vi "Incorporate New Data.vi"(8 "error in (no error)":cluster{"状态":bool, "代码":i32, "源":string} caption="错误输入（无错误）", 10 "新图形数据":waveform(dbl)[](array[waveform]), 11 "数据输入":T1={"UI引用"={"退出引用"=refnum, "保存引用"=refnum, "打开引用"=refnum, "导出引用"=refnum, "采集引用"=refnum, "配置引用"=refnum, "图形引用"=refnum, "清空引用"=refnum, "分析引用"=refnum, "状态引用"=refnum, "快照引用"=refnum}, "图形数据"={"数据"=[], "注释列表"=[], "游标列表"=[], "分析数据"=[]}, "用户定义"={"硬件配置"={"硬件引用句柄<替换此项>"="", "信号类型<替换该项>"=enum."Sine Wave"}, "分析配置"={"统计"=TRUE}, "新采集到数据时如何操作"=enum."Replace"}}) -> (0 "error out":cluster{"状态":bool, "代码":i32, "源":string} caption="错误输出", 3 "数据输出":T1={"UI引用"={"退出引用"=refnum, "保存引用"=refnum, "打开引用"=refnum, "导出引用"=refnum, "采集引用"=refnum, "配置引用"=refnum, "图形引用"=refnum, "清空引用"=refnum, "分析引用"=refnum, "状态引用"=refnum, "快照引用"=refnum}, "图形数据"={"数据"=[], "注释列表"=[], "游标列表"=[], "分析数据"=[]}, "用户定义"={"硬件配置"={"硬件引用句柄<替换此项>"="", "信号类型<替换该项>"=enum."Sine Wave"}, "分析配置"={"统计"=TRUE}, "新采集到数据时如何操作"=enum."Replace"}})   [LabVIEW 2022 SP3]
doc: "将新采集到的数据或加载的数据与主状态数据整合。 新数据可以替换、追加，或与原有数据重叠（作为额外的通道）。 如尚无保存好的用户配置，将会弹出对话框询问用户。"
uses:
  controls/Data.ctl
  controls/UI References.ctl
  controls/Graph Data.ctl
  <vilib>/Utility/miscctls.llb/LVAnnotationListTypeDef.ctl
  <vilib>/Utility/miscctls.llb/LVCursorListTypeDef.ctl
  controls/User Specified Data.ctl
  controls/HW Configuration.ctl
  controls/Simulated Signal Type.ctl
  controls/Analysis Configuration.ctl
  controls/New Data Behavior.ctl
panel:
  # "（向上滚动可查看大型状态数据输入/输出簇）"
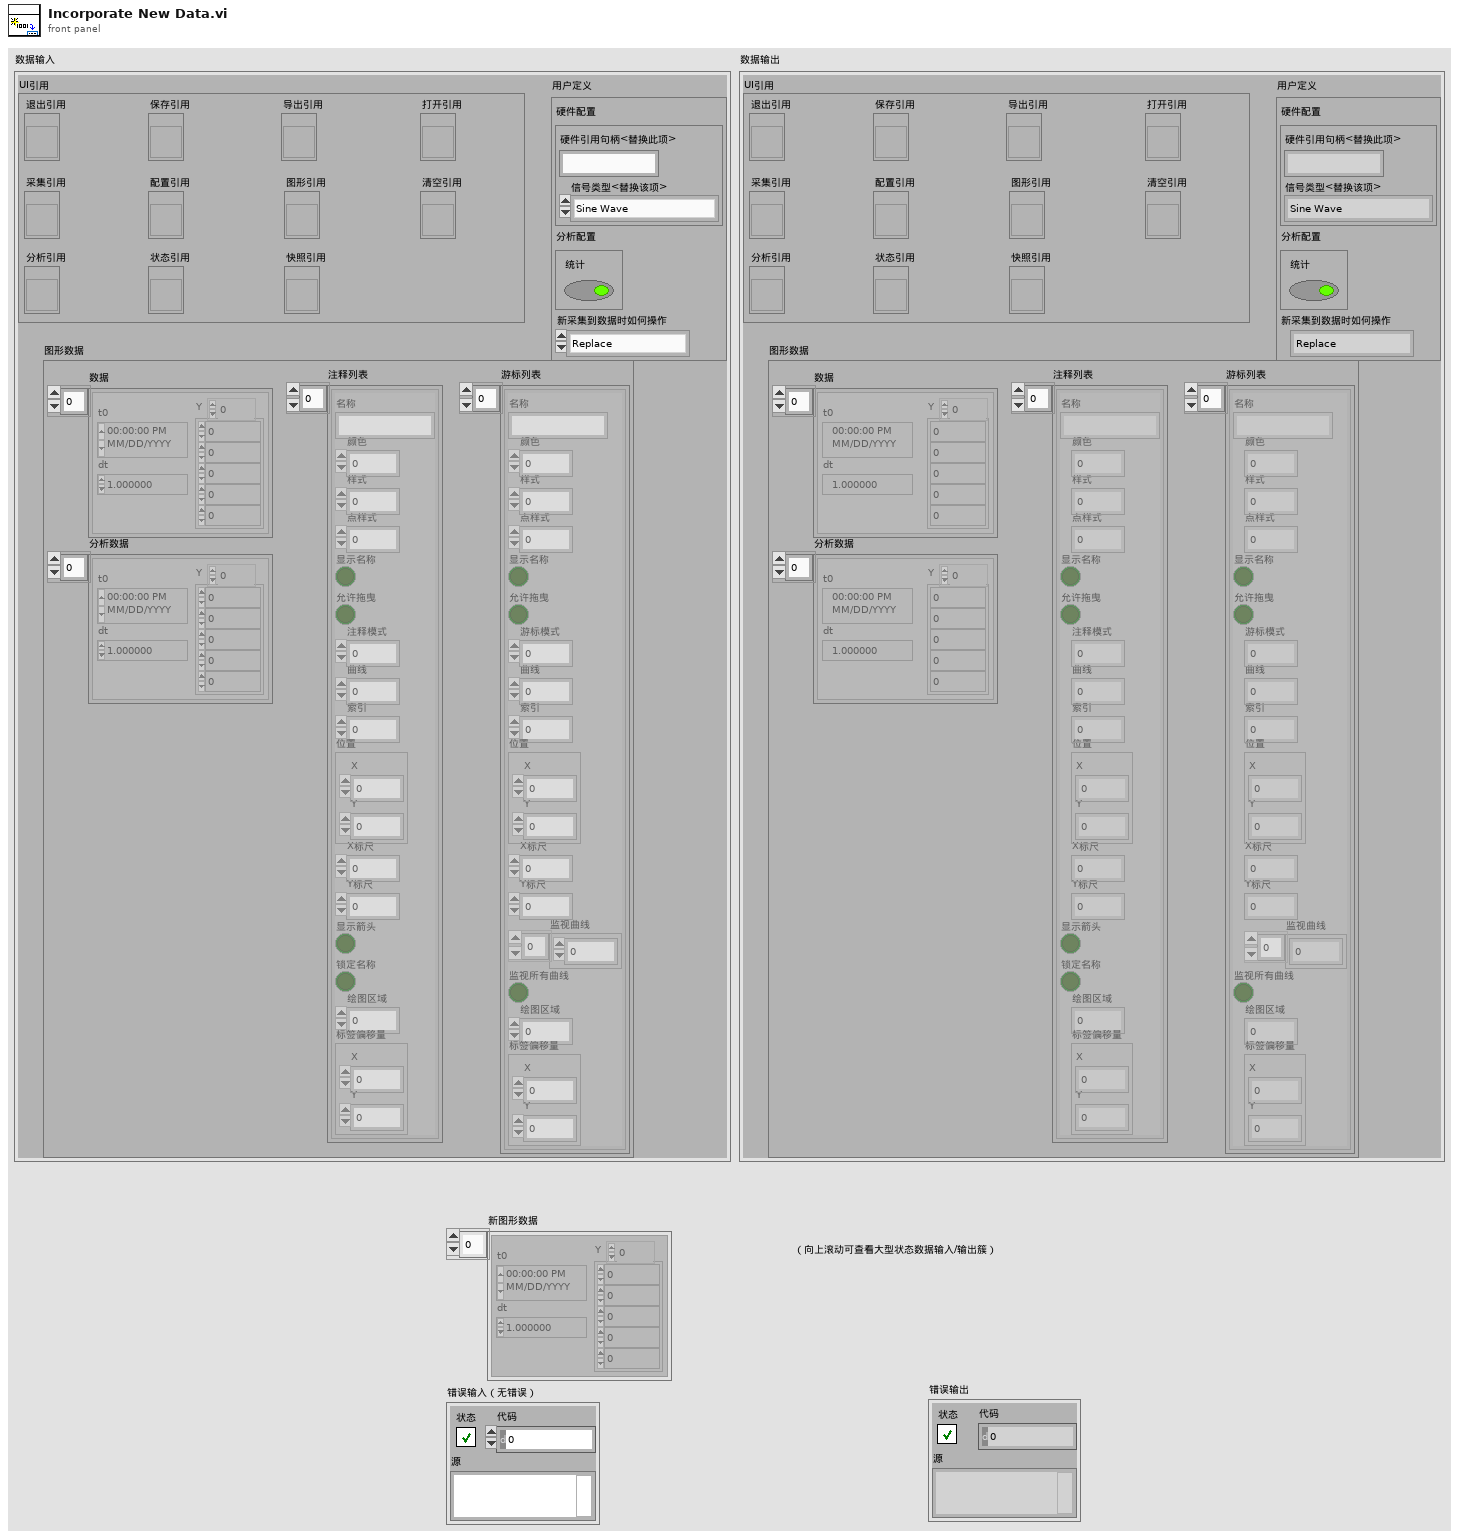
[diagram p1: front panel]
types:
  T1 = typedef "Data.ctl" = cluster{"UI引用":T2, "图形数据":T3, "用户定义":T6}
  T2 = typedef "UI References.ctl" = cluster{"退出引用":refnum<vi>, "保存引用":refnum<vi>, "打开引用":refnum<vi>, "导出引用":refnum<vi>, "采集引用":refnum<vi>, "配置引用":refnum<vi>, "图形引用":refnum<vi>, "清空引用":refnum<vi>, "分析引用":refnum<vi>, "状态引用":refnum<vi>, "快照引用":refnum<vi>}
  T3 = typedef "Graph Data.ctl" = cluster{"数据":waveform(dbl)[], "注释列表":T4, "游标列表":T5, "分析数据":waveform(dbl)[]}
  T4 = typedef "LVAnnotationListTypeDef.ctl" = cluster{"Name":string, "Color":u32, "Style":u8, "Point Style":u8, "Name Visible":bool, "Allow Drag":bool, "Annotation Mode":u32, "Plot":i32, "Index":i32, "Position":cluster{"X":dbl, "Y":dbl}, "X Scale":u32, "Y Scale":u32, "Show Arrow":bool, "Lock Name":bool, "Plot Area":i32, "Label Offset":cluster{"X":dbl, "Y":dbl}}[]
  T5 = typedef "LVCursorListTypeDef.ctl" = cluster{"Name":string, "Color":u32, "Style":u8, "Point Style":u8, "Name Visible":bool, "Allow Drag":bool, "Cursor Mode":u32, "Plot":i32, "Index":i32, "Position":cluster{"X":dbl, "Y":dbl}, "X Scale":u32, "Y Scale":u32, "Watch Plots":i32[], "Watch All Plots":bool, "Plot Area":i32, "Label Offset":cluster{"X":dbl, "Y":dbl}}[]
  T6 = typedef "User Specified Data.ctl" = cluster{"硬件配置":T7, "分析配置":T9, "新采集到数据时如何操作":T10}
  T7 = typedef "HW Configuration.ctl" = cluster{"硬件引用句柄<替换此项>":string, "信号类型<替换该项>":T8}
  T8 = typedef "Simulated Signal Type.ctl" = enum16{"Sine Wave", "Square Wave"}
  T9 = typedef "Analysis Configuration.ctl" = cluster{"统计":bool}
  T10 = typedef "New Data Behavior.ctl" = enum16{"Replace", "Overlay", "Append"}
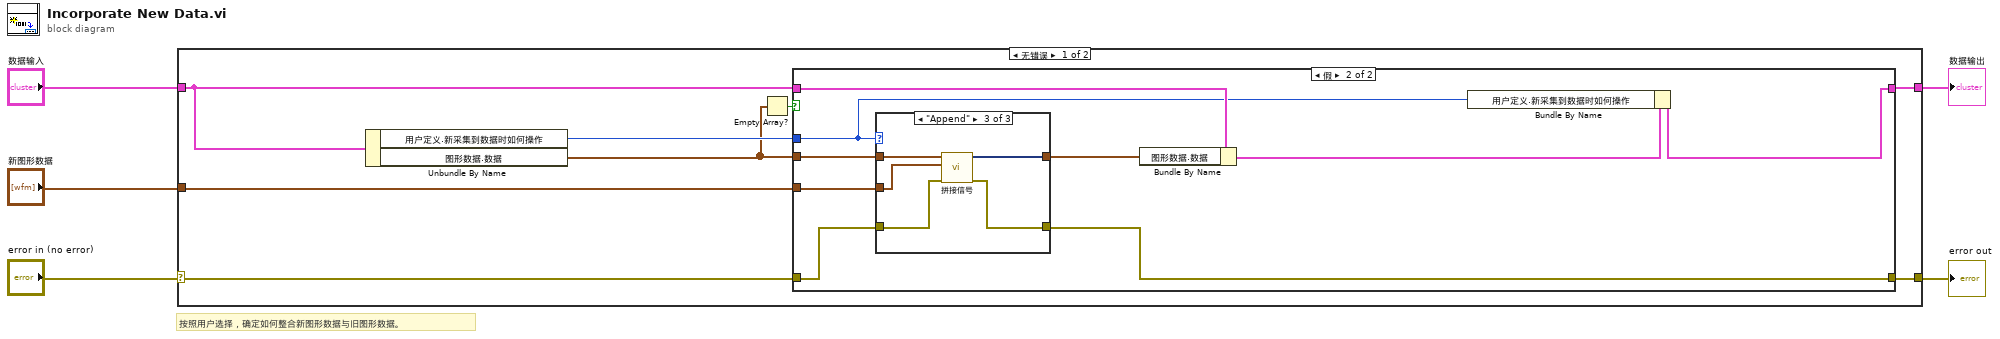
[diagram p0: block diagram]
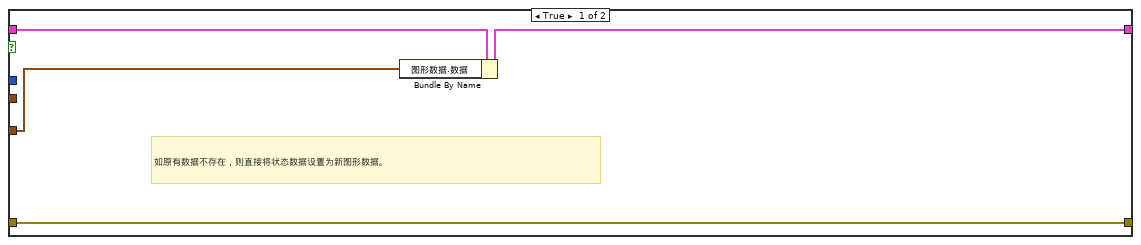
[diagram p2: hidden frame]
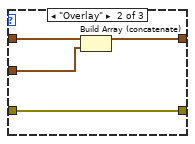
[diagram p4: hidden frame]
diagram:
  # "按照用户选择，确定如何整合新图形数据与旧图形数据。"
  n1 = case shown="无错误" "error in (no error)" {
    selector: "error in (no error)" -> [w9 w39]
    tunnel: "数据输入" -> [w13 w38]
    tunnel: "新图形数据" -> [w11 _]
    tunnel: [w10 w38] -> w3
    tunnel: [w8 w39] -> w1
    frame No Error {
      n2 = Unbundle By Name(w13) -> ("用户定义.新采集到数据时如何操作"=w12:T10, "图形数据.数据"=w7:waveform(dbl)[])
      n3 = Empty Array?(array=w7) -> (empty?=w6:bool)
      n4 = case shown="假" w6 {
        tunnel: w13 -> [w17 w26]
        tunnel: w12 -> [_ w18]
        tunnel: w11 -> [w16 w25]
        tunnel: w7 -> [_ w23]
        tunnel: [w15 w21] -> w10
        tunnel: w9 -> [w14 w20]
        tunnel: [w14 w19] -> w8
        frame True {
          # "如原有数据不存在，则直接将状态数据设置为新图形数据。"
          n5 = Bundle By Name(cluster=w17, "图形数据.数据"=w16) -> (w15:T1)
        }
        frame False {
          n6 = case shown="\"Append\"" w18 {
            tunnel: w25 -> [w28 w31 w36]
            tunnel: [w28 w30 w35] -> w24
            tunnel: w23 -> [_ w32 w37]
            tunnel: w20 -> [w27 w29 w34]
            tunnel: [w27 w29 w33] -> w19
            frame "Replace" {
            }
            frame "Overlay" {
              n7 = Build Array (concatenate)(w32, w31) -> (w30:waveform(dbl)[])
            }
            frame "Append" {
              n8 = call "拼接信号"("error in (no error)"=w34, "Input Signal B"=w36, "Input Signal A"=w37) -> ("error out"=w33:errorcluster, "Appended Signals"=w35:dynamicdata)  [unwired: 7 in]
            }
          }
          n9 = Bundle By Name(cluster=w26, "图形数据.数据"=w24) -> (w22:T1)
          n10 = Bundle By Name(cluster=w22, "用户定义.新采集到数据时如何操作"=w18) -> (w21:T1)
        }
      }
    }
    frame Error {
    }
  }
  "数据输出" <- w3
  "error out" <- w1
